vi "split array.vi"(2 "string":string, 4 "char (,)":string=",") -> (7 "split arr":string[](array[string]))   [LabVIEW 2013, in "CreateOPCUAServerAuto.lvlib"]
uses:
  CreateOPCUAServerAuto.lvlib
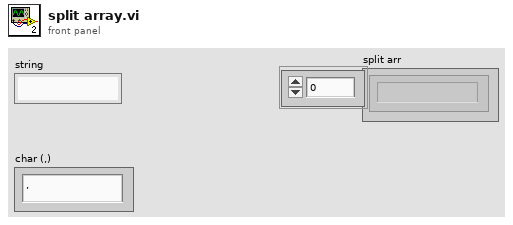
[diagram p1: front panel]
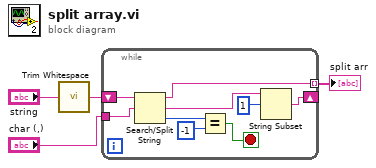
[diagram p0: block diagram]
diagram:
  n1 = call <vilib>:"Trim Whitespace.vi"("string"="string") -> ("trimmed string"=w4:string)  [unwired: 1 in]
  n2 = while {
    shift-right: [w7] -> _
    shift-left: w4 -> [w12]
    tunnel: [w13] -> w2 mode=indexing
    tunnel: "char (,)" -> [w5]
    stop <- w9 stop-if-true
    n3 = Search/Split String(string=w12, search string/char (-)=w5) -> (substring before match=w13:string, match + rest of string=w8:string, offset of match=w11:i32)  [unwired: 1 in]
    n4 = Equal?(x=w11, y=-1) -> (x = y?=w9:bool)
    n5 = String Subset(string=w8, offset (0)=1) -> (substring=w7:string)  [unwired: 1 in]
  }
  "split arr" <- w2
